vi "Initialize.vi"(8 "error in (no error)":errorcluster, 9 "Channel":i32, 10 "VISA resource name":refnum<visa-resource-name>="COM8", 11 "YP03-60_Y in":refnum<class "YP03-60_Y.lvclass">) -> (0 "error out":errorcluster, 3 "YP03-60_Y out":refnum<class "YP03-60_Y.lvclass">)   [LabVIEW 2020, in "PowerControl.lvlib" / "YP03-60_Y.lvclass"]
uses:
  YP03-60_Y.lvclass
  YP03-60_X/YP03-60_X.lvclass
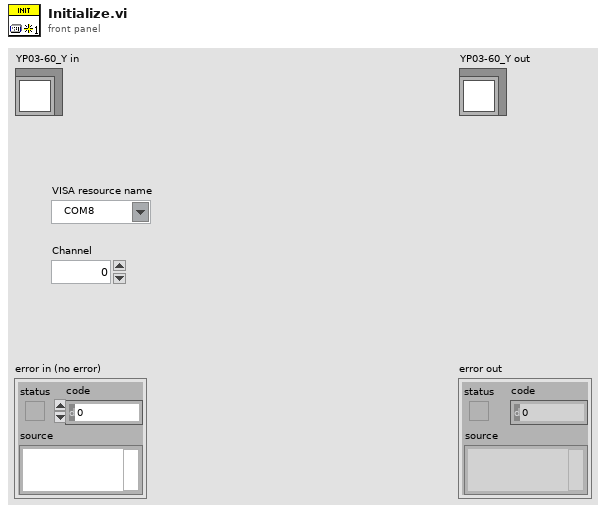
[diagram p1: front panel]
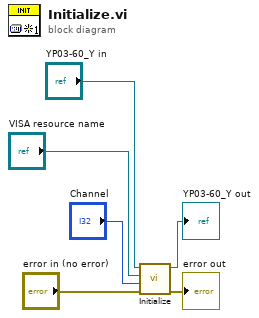
[diagram p0: block diagram]
diagram:
  n1 = call-parent "Initialize.vi"("error in (no error)"="error in (no error)", "Channel"="Channel", "VISA resource name"="VISA resource name", "YP03-60_X in"="YP03-60_Y in") -> ("error out"=→"error out":errorcluster, "YP03-60_X out"=→"YP03-60_Y out":refnum<class "YP03-60_Y.lvclass">)  [unwired: 6 in]
